vi "Move Mouse.vi"(8 "error in (no error)":errorcluster, 9 "Board Game in":refnum<class "Board Game.lvclass">, 10 "Packed refs":T1, 11 "Mouse in":refnum<class "Mouse.lvclass">) -> (0 "error out":errorcluster, 3 "Mouse out":refnum<class "Mouse.lvclass">)   [LabVIEW 2021, in "Mouse.lvclass"]
uses:
  Mouse.lvclass
  C:/Users/poche/Programs/LabVIEW/imposible snake/GameEl_class/GameEl.lvclass
  Board Game_class/Board Game.lvclass
  Application/Packed Refs.ctl
  GameEl_class/private/Enum Direction.ctl
  LVApp/Modules/Sound Manager/Typedefs/Sound Effects.ctl
  Mouse.lvclass/Mouse.ctl
  GameEl_class/GameEl.lvclass/GameEl.ctl
  Board Game_class/Board Game.lvclass/Board Game.ctl
  Snake_class/Read Snake Head.vi
  Board Game_class/Read Snake.vi
  GameEl_class/Read position.vi
  Read Init Mouse.vi
  Snake_class/Snake.lvclass
  GameEl_class/GameEl.lvclass
  Application/Application.lvclass
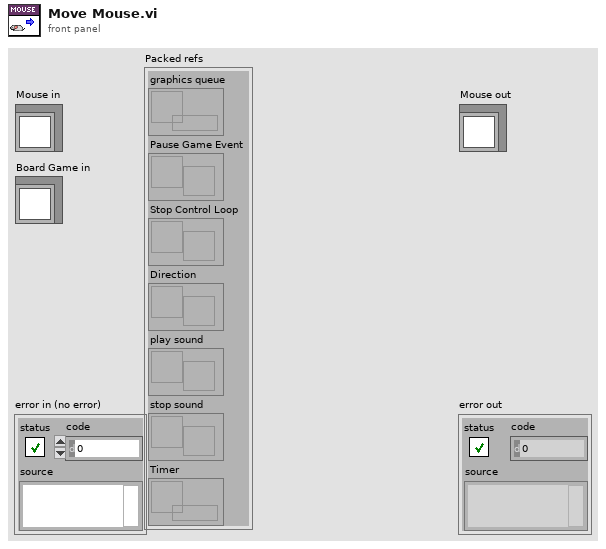
[diagram p1: front panel]
types:
  T1 = typedef "Application.lvclass/Packed Refs.ctl" = cluster{"graphics queue":refnum<queue>, "Pause Game Event":refnum<user-event>, "Stop Control Loop":refnum<user-event>, "Direction":refnum<notifier>, "play sound":refnum<user-event>, "stop sound":refnum<user-event>, "Timer":refnum<data-value>}
  T2 = typedef "GameEl.lvclass/Enum Direction.ctl" = enum16{"Up", "Down", "Forward", "Backward"}
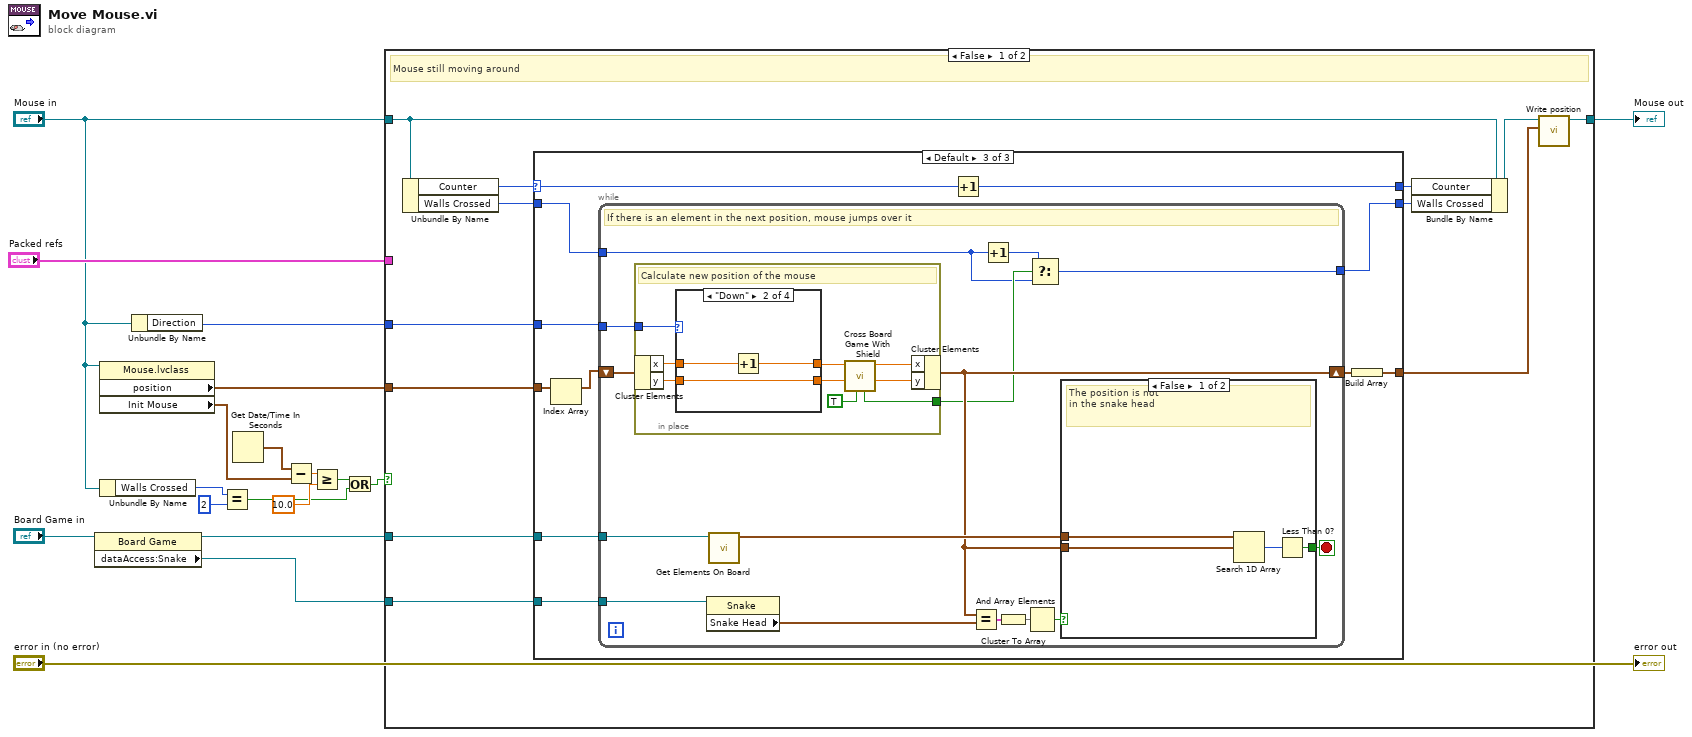
[diagram p0: block diagram]
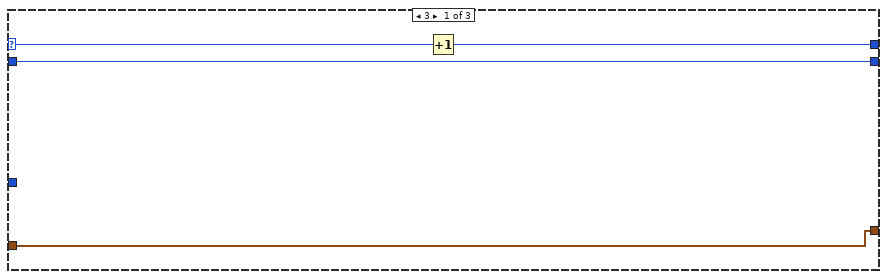
[diagram p2: hidden frame]
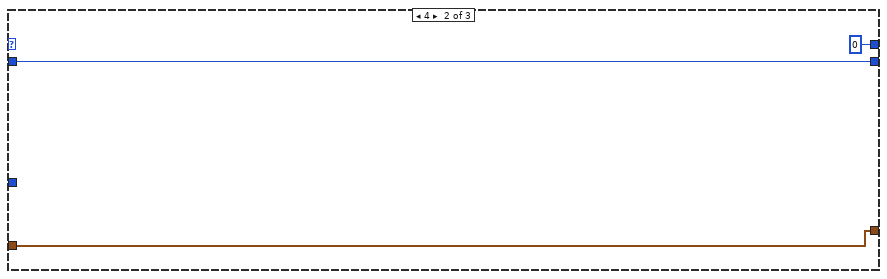
[diagram p3: hidden frame]
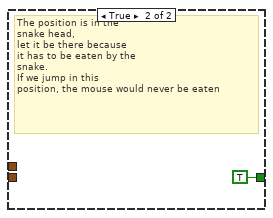
[diagram p4: hidden frame]
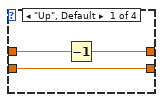
[diagram p5: hidden frame]
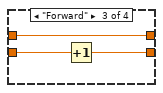
[diagram p6: hidden frame]
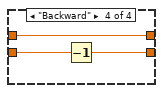
[diagram p7: hidden frame]
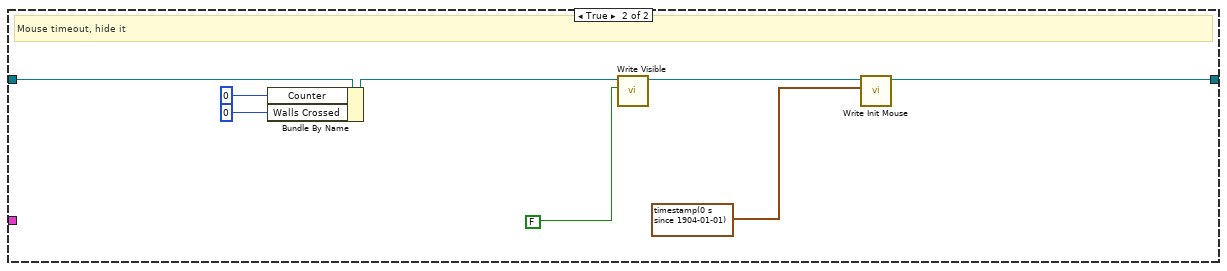
[diagram p8: hidden frame]
diagram:
  n1 = property class="Board Game"(reference="Board Game in") -> (reference out=w13:refnum<class "Board Game.lvclass">, "dataAccess:Snake"=w12:refnum<class "Snake.lvclass">)  [unwired: 1 in, 1 out]
  n2 = property class="Mouse.lvclass"(reference="Mouse in") -> ("position"=w16:cluster{"x":dbl, "y":dbl}[], "Init Mouse"=w11:timestamp)  [unwired: 1 in, 2 out]
  n3 = Unbundle By Name("Mouse in") -> ("Walls Crossed"=w4:u32)
  n4 = Unbundle By Name("Mouse in") -> ("Direction"=w17:T2)
  n5 = Equal?(x=w4, y=u32 2) -> (x = y?=w1:bool)
  n6 = Get Date/Time In Seconds() -> (seconds since 1Jan1904=w10:timestamp)
  n7 = Subtract(x=w10, y=w11) -> (x-y=w9:dbl)
  n8 = Greater Or Equal?(x=w9, y=10.0) -> (x >= y?=w7:bool)
  n9 = Or(x=w7, y=w1) -> (x .or. y?=w2:bool)
  n10 = case shown="False" w2 {
    tunnel: w17 -> [w30 _]
    tunnel: "Mouse in" -> [w24 w97]
    tunnel: w16 -> [w29 _]
    tunnel: [w28 w94] -> w15
    tunnel: w13 -> [w26 _]
    tunnel: w12 -> [w25 _]
    tunnel: "Packed refs" -> [_ _]
    frame False {
      # "Mouse still moving around"
      n11 = Unbundle By Name(w24) -> ("Counter"=w22:u32, "Walls Crossed"=w20:u32)
      n12 = case shown="Default" w22 {
        selector: w22 -> [w33 _ w41]
        tunnel: w30 -> [_ _ w48]
        tunnel: w29 -> [w34 w37 w47]
        tunnel: [w34 w37 w44] -> w27
        tunnel: w26 -> [_ _ w43]
        tunnel: w25 -> [_ _ w42]
        tunnel: [w32 u32 0 w40] -> w21
        tunnel: w20 -> [w31 w35 w39]
        tunnel: [w31 w35 w38] -> w19
        frame 3 {
          n13 = Increment(x=w33) -> (x+1=w32:u32)
        }
        frame 4 {
        }
        frame Default {
          n14 = Index Array(array=w47) -> (element=w46:cluster{"x":dbl, "y":dbl})  [unwired: 1 in]
          n15 = while {
            tunnel: w48 -> [w63]
            tunnel: w43 -> [w61]
            shift-right: [w56] -> w45
            shift-left: w46 -> [w62]
            tunnel: w42 -> [w58]
            tunnel: w39 -> [w50]
            tunnel: [w49] -> w38
            stop <- w59 stop-if-true
            # "If there is an element in the next position, mouse jumps over it"
            n16 = in-place {
              in-place-border: w63 -> [w77]
              in-place-border: [w69] -> w52
              # "Calculate new position of the mouse"
              n17 = in-place-cluster #1(w62) -> ("x"=w76:dbl, "y"=w75:dbl)
              n18 = case shown="\"Down\"" w77 {
                tunnel: w76 -> [w80 w83 w86 w89]
                tunnel: w75 -> [w79 w82 w85 w88]
                tunnel: [w78 w81 w86 w89] -> w74
                tunnel: [w79 w82 w84 w87] -> w73
                frame "Up", Default {
                  n19 = Decrement(x=w80) -> (x-1=w78:dbl)
                }
                frame "Down" {
                  n20 = Increment(x=w83) -> (x+1=w81:dbl)
                }
                frame "Forward" {
                  n21 = Increment(x=w85) -> (x+1=w84:dbl)
                }
                frame "Backward" {
                  n22 = Decrement(x=w88) -> (x-1=w87:dbl)
                }
              }
              n23 = call "Cross Board Game With Shield.vi"("Max Shield?"=TRUE, "y"=w73, "x"=w74) -> ("y out"=w71:dbl, "x out"=w72:dbl, "Crossed?"=w69:bool)  [unwired: 6 in]
              n24 = in-place-cluster #1("x"=w72, "y"=w71) -> (w56:cluster{"x":dbl, "y":dbl})
            }
            n25 = property class="Snake"(reference=w58) -> ("Snake Head"=w57:cluster{"x":dbl, "y":dbl})  [unwired: 1 in, 2 out]
            n26 = call "Get Elements On Board.vi"("Board Game in"=w61) -> ("position"=w60:cluster{"x":dbl, "y":dbl}[])  [unwired: 9 in, 1 out]
            n27 = Equal?(x=w56, y=w57) -> (x = y?=w55:cluster{"x":bool, "y":bool})
            n28 = Increment(x=w50) -> (x+1=w51:u32)
            n29 = Cluster To Array(cluster=w55) -> (array=w54:bool[])
            n30 = And Array Elements(Boolean array=w54) -> (logical AND=w53:bool)
            n31 = Select(t=w51, s=w52, f=w50) -> (s? t:f=w49:u32)
            n32 = case shown="False" w53 {
              tunnel: w60 -> [w67 _]
              tunnel: [w65 TRUE] -> w59
              tunnel: w56 -> [w64 _]
              frame False {
                # "The position is not \nin the snake head"
                n33 = Search 1D Array(1D array=w67, element=w64) -> (index of element=w66:i32)  [unwired: 1 in]
                n34 = Less Than 0?(x=w66) -> (x < 0?=w65:bool)
              }
              frame True {
                # "The position is in the \nsnake head, \nlet it be there because\nit has to be eaten by the \nsnake. \nIf we jump in this \nposition, the mouse would never be eaten"
              }
            }
          }
          n35 = Increment(x=w41) -> (x+1=w40:u32)
          n36 = Build Array(w45) -> (w44:cluster{"x":dbl, "y":dbl}[])
        }
      }
      n37 = Bundle By Name(cluster=w24, "Counter"=w21, "Walls Crossed"=w19) -> (w23:refnum<class "Mouse.lvclass">)
      n38 = call "Write position.vi"("position"=w27, "GameEl in"=w23) -> ("GameEl out"=w28:refnum<class "Mouse.lvclass">)  [unwired: 8 in, 1 out]
    }
    frame True {
      # "Mouse timeout, hide it"
      n39 = Bundle By Name(cluster=w97, "Counter"=u32 0, "Walls Crossed"=u32 0) -> (w92:refnum<class "Mouse.lvclass">)
      n40 = call "Write Visible.vi"("Visible"=FALSE, "GameEl in"=w92) -> ("GameEl out"=w96:refnum<class "Mouse.lvclass">)  [unwired: 8 in, 1 out]
      n41 = call "Write Init Mouse.vi"("Init Mouse"=timestamp(0 s since 1904-01-01), "Mouse in"=w96) -> ("Mouse out"=w94:refnum<class "Mouse.lvclass">)  [unwired: 8 in, 1 out]
    }
  }
  "Mouse out" <- w15
  "error out" <- "error in (no error)"
